vi "Finish.vi"   [LabVIEW 2013]
doc: "This VI is called just before exiting. It is expected to close I/O refnum, save collected data, etc."
uses:
  <vilib>/Rock Robotics/WPI/Compressor/WPI_CompressorGetSetRefNum.vi
  <vilib>/Rock Robotics/WPI/Joystick/WPI_JoystickGetSetRefNum.vi
  <vilib>/Rock Robotics/WPI/RobotDrive/WPI_RobotDriveGetSetRefNum.vi
types:
  T1 = typedef "WPI_JoystickDevRef.ctl" = cluster{"Device":T2}
  T2 = typedef "WPI_JoystickDeviceEnum.ctl" = enum16{"USB 1", "USB 2", "USB 3", "USB 4", "Kinect 1", "Kinect 2"}
  T3 = typedef "WPI_MotorControlDeviceRef.ctl" = cluster{"DeviceStatus":errorcluster, "Type":enum16{"PWM", "CAN"}, "PWM":cluster{"Digital Module":T4, "PWM Channel":T5, "DeadBand":T6}, "CAN":cluster{"Device Number":u8, "Control Mode":T7, "Semaphore":T8, "Max Vout":dbl}, "Invert":bool, "TransformRef":T9, "InvTransformRef":T9}
  T4 = typedef "FPGA_TypedefDigitalModule.ctl" = enum16{"Digital Module 1", "Digital Module 2"}
  T5 = typedef "FPGA_DIOPWMChannel.ctl" = enum8{"PWM 1", "PWM 2", "PWM 3", "PWM 4", "PWM 5", "PWM 6", "PWM 7", "PWM 8", "PWM 9", "PWM 10", "Invalid"}
  T6 = typedef "WPI_PWMDeadband.ctl" = cluster{"Name":string, "maxPositivePwm":i32, "minPositivePwm":i32, "centerPwm":i32, "maxNegativePwm":i32, "minNegativePwm":i32, "angularRange":u16}
  T7 = typedef "WPI_CANJaguar_ControlMode.ctl" = enum8{"Percent VBus", "Current", "Speed", "Position", "Voltage"}
  T8 = typedef "Semaphore RefNum" = refnum<k1>
  T9 = typedef "WPI_PWMTransform_ConPane.ctl" = refnum<vi>
  T10 = typedef "WPI_CompressorDevRef.ctl" = cluster{"DevStatus":errorcluster, "DigitalInputDevRef":T11, "RelayDevRef":T13}
  T11 = typedef "WPI_DigitalInputDevRef.ctl" = cluster{"DevStatus":errorcluster, "DIO Channel":T12, "Digital Module":T4}
  T12 = typedef "FPGA_DIOChannel.ctl" = enum8{"DIO 1", "DIO 2", "DIO 3", "DIO 4", "DIO 5", "DIO 6", "DIO 7", "DIO 8", "DIO 9", "DIO 10", "DIO 11", "DIO 12", "DIO 13", "DIO 14", "Invalid"}
  T13 = typedef "WPI_RelayDevRef.ctl" = cluster{"DevStatus":errorcluster, "Relay Channel":T14, "Digital Module":T4, "Relay Direction":T15}
  T14 = typedef "FPGA_DIORelayChannel.ctl" = enum8{"Relay 1", "Relay 2", "Relay 3", "Relay 4", "Relay 5", "Relay 6", "Relay 7", "Relay 8", "Invalid"}
  T15 = typedef "WPI_RelayDirection.ctl" = enum16{"Both directions", "Forward only", "Reverse only"}
  T16 = typedef "WPI_AnalogChannelDevRef.ctl" = cluster{"DevStatus":errorcluster, "Analog Module":T17, "Analog Channel":T18}
  T17 = typedef "FPGA_TypedefAnalogModule.ctl" = enum16{"Analog Module 1", "Analog Module 2"}
  T18 = typedef "FPGA_AIChannel.ctl" = enum8{"AI 1", "AI 2", "AI 3", "AI 4", "AI 5", "AI 6", "AI 7", "AI 8", "Invalid"}
  T19 = typedef "WPI_SolenoidDevRef.ctl" = cluster{"DevStatus":errorcluster, "Solenoid Module":T20, "Forward Solenoid Channel":T21, "Reverse Solenoid Channel":T21}
  T20 = typedef "FPGA_TypedefSolenoidModule.ctl" = enum16{"Solenoid Module 1", "Solenoid Module 2"}
  T21 = typedef "WPI_SolenoidChannel.ctl" = enum8{"Solenoid 1", "Solenoid 2", "Solenoid 3", "Solenoid 4", "Solenoid 5", "Solenoid 6", "Solenoid 7", "Solenoid 8", "Invalid"}
  T22 = typedef "WPI_RobotDriveDevRef.ctl" = cluster{"DevStatus":errorcluster, "Motors[]":T3[], "Square Inputs":bool, "Max Output":dbl, "Isochronous":bool}
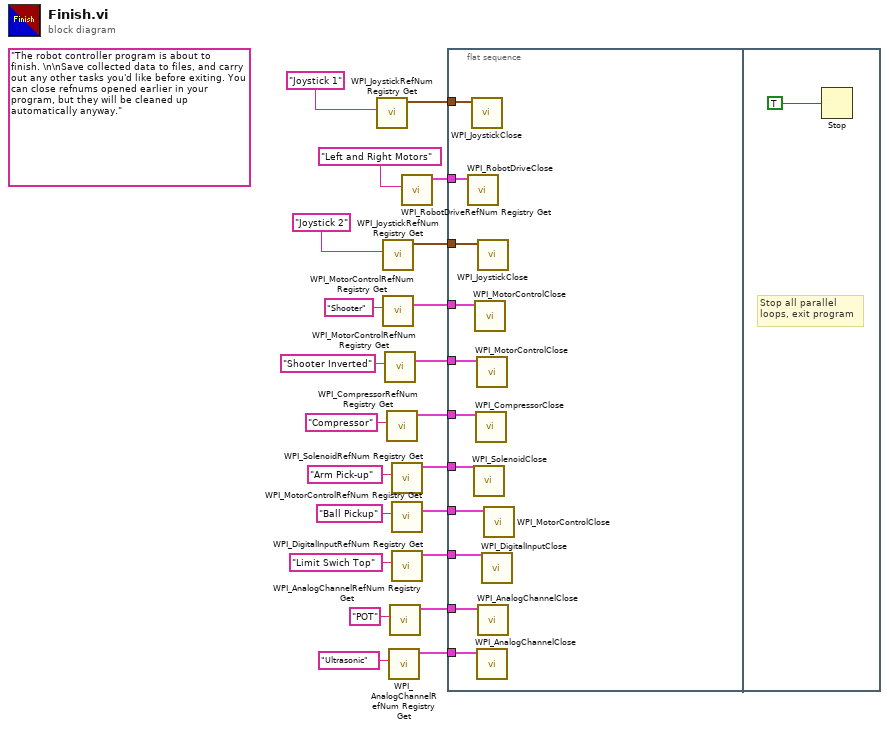
[diagram p0: block diagram]
diagram:
  (unwired) "The robot controller program is about to finish. \n\nSave collected data to files, and carry out any other tasks you'd like before exiting. You can close refnums opened earlier in your program, but they will be cleaned up automatically anyway."
  n1 = call <vilib>:"WPI_JoystickRefNum Registry Get.vi"("refnum name"="Joystick 1") -> ("JoystickDevRef"=w19:T1)  [unwired: 1 in, 9 out]
  n2 = call <vilib>:"WPI_JoystickRefNum Registry Get.vi"("refnum name"="Joystick 2") -> ("JoystickDevRef"=w18:T1)  [unwired: 1 in, 9 out]
  n3 = call <vilib>:"WPI_MotorControlRefNum Registry Get.vi"("refnum name"="Shooter") -> ("MotorControlDevRef"=w15:T3)  [unwired: 9 in, 1 out]
  n4 = call <vilib>:"WPI_MotorControlRefNum Registry Get.vi"("refnum name"="Shooter Inverted") -> ("MotorControlDevRef"=w14:T3)  [unwired: 9 in, 1 out]
  n5 = call <vilib>:"WPI_CompressorRefNum Registry Get.vi"("refnum name"="Compressor") -> ("CompressorDevRef"=w11:T10)  [unwired: 9 in, 1 out]
  n6 = call <vilib>:"WPI_AnalogChannelRefNum Registry Get.vi"("refnum name"="Ultrasonic") -> ("AIDeviceRef"=w1:T16)  [unwired: 9 in, 1 out]
  n7 = call <vilib>:"WPI_AnalogChannelRefNum Registry Get.vi"("refnum name"="POT") -> ("AIDeviceRef"=w4:T16)  [unwired: 9 in, 1 out]
  n8 = call <vilib>:"WPI_SolenoidRefNum Registry Get.vi"("refnum name"="Arm Pick-up") -> ("SolenoidDevRef"=w9:T19)  [unwired: 9 in, 1 out]
  n9 = call <vilib>:"WPI_MotorControlRefNum Registry Get.vi"("refnum name"="Ball Pickup") -> ("MotorControlDevRef"=w8:T3)  [unwired: 9 in, 1 out]
  n10 = call <vilib>:"WPI_DigitalInputRefNum Registry Get.vi"("refnum name"="Limit Swich Top") -> ("DigitalInputDevRef"=w6:T11)  [unwired: 9 in, 1 out]
  n11 = call <vilib>:"WPI_RobotDriveRefNum Registry Get.vi"("refnum name"="Left and Right Motors") -> ("RobotDriveDevRef"=w20:T22)  [unwired: 1 in, 9 out]
  n12 = flat-sequence {
    tunnel: w20 -> [w33]
    tunnel: w19 -> [w32]
    tunnel: w18 -> [w31]
    tunnel: w15 -> [w30]
    tunnel: w14 -> [w29]
    tunnel: w11 -> [w28]
    tunnel: w9 -> [w27]
    tunnel: w8 -> [w26]
    tunnel: w6 -> [w25]
    tunnel: w4 -> [w24]
    tunnel: w1 -> [w23]
    frame #0 {
      n13 = call <vilib>:"WPI_RobotDriveClose.vi"("RobotDriveDevRef"=w33) -> ()  [unwired: 1 in, 10 out]
      n14 = call <vilib>:"WPI_JoystickClose.vi"("JoystickDevRef"=w32) -> ()  [unwired: 11 out]
      n15 = call <vilib>:"WPI_SolenoidClose.vi"("SolenoidDevRef"=w27) -> ()  [unwired: 10 in, 1 out]
      n16 = call <vilib>:"WPI_MotorControlClose.vi"("MotorControlDevRef"=w30) -> ()  [unwired: 10 in, 1 out]
      n17 = call <vilib>:"WPI_CompressorClose.vi"("CompressorDevRef"=w28) -> ()  [unwired: 10 in, 1 out]
      n18 = call <vilib>:"WPI_MotorControlClose.vi"("MotorControlDevRef"=w29) -> ()  [unwired: 10 in, 1 out]
      n19 = call <vilib>:"WPI_AnalogChannelClose.vi"("AIDeviceRef"=w23) -> ()  [unwired: 10 in, 1 out]
      n20 = call <vilib>:"WPI_JoystickClose.vi"("JoystickDevRef"=w31) -> ()  [unwired: 11 out]
      n21 = call <vilib>:"WPI_AnalogChannelClose.vi"("AIDeviceRef"=w24) -> ()  [unwired: 10 in, 1 out]
      n22 = call <vilib>:"WPI_DigitalInputClose.vi"("DigitalInputDevRef"=w25) -> ()  [unwired: 10 in, 1 out]
      n23 = call <vilib>:"WPI_MotorControlClose.vi"("MotorControlDevRef"=w26) -> ()  [unwired: 10 in, 1 out]
    }
    frame #1 {
      # "Stop all parallel\nloops, exit program"
      n24 = Stop(stop? (T)=TRUE ("Quit")) -> ()
    }
  }
